vi "UpdateTree(SingleLine).vi"(7 "New Item Indentation":i32, 8 "error in (no error)":errorcluster, 9 "Item Properties":string[](array[string]), 10 "Item Name":string, 11 "Tree Reference":refnum<vi>) -> (0 "error out":errorcluster)   [LabVIEW 2017, in "Client.lvlib" / "UI_API.lvlib"]
uses:
  UI_API.lvlib
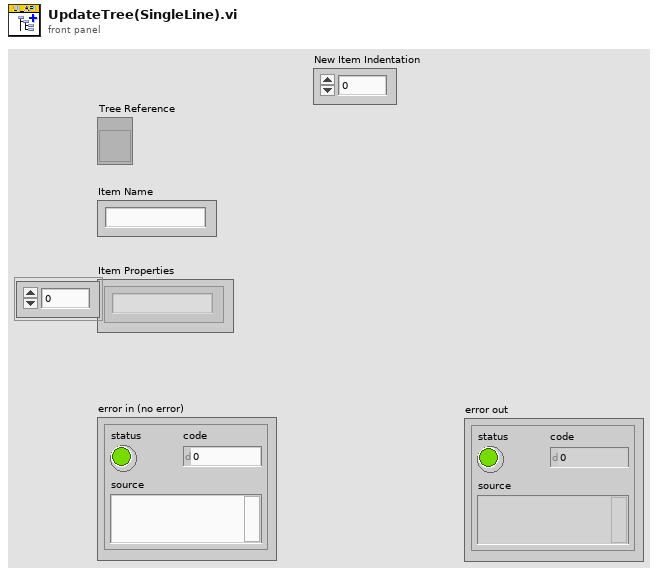
[diagram p1: front panel]
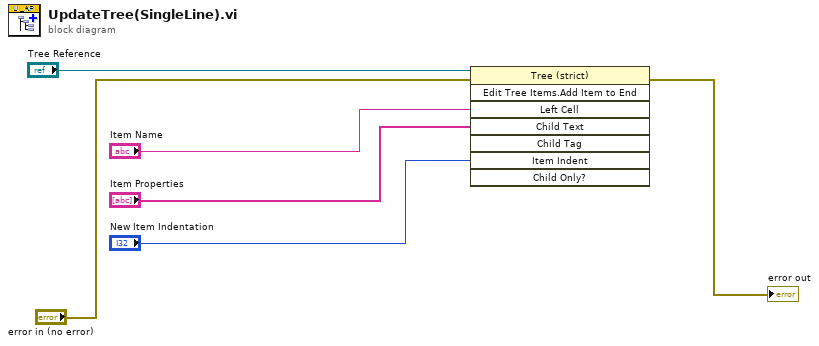
[diagram p0: block diagram]
diagram:
  n1 = invoke on="Invoke Node" class="Tree (strict)" method="Edit Tree Items.Add Item to End"(reference="Tree Reference", error in="error in (no error)", "Left Cell"="Item Name", "Child Text"="Item Properties", "Item Indent"="New Item Indentation") -> (error out=→"error out":errorcluster)  [unwired: 3 in, 7 out]
